vi "camera mjpeg.vi"(11 "CameraDevRef":T1) -> ()   [LabVIEW 2013]
uses:
  <vilib>/Rock Robotics/WPI/Camera/WPI_CameraDevRef.ctl
  <vilib>/Rock Robotics/WPI/Camera/WPI_CameraSettings Operations.ctl
  typedefs/fg_getset.ctl
  typedefs/vision/vision enable.ctl
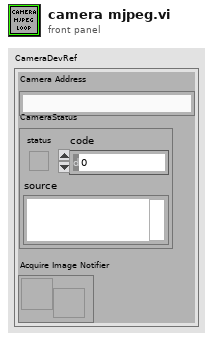
[diagram p1: front panel]
types:
  T1 = typedef "WPI_CameraDevRef.ctl" = cluster{"Camera Address":string, "CameraStatus":errorcluster, "Acquire Image Notifier":refnum<notifier>}
  T2 = typedef "WPI_CameraSettings Operations.ctl" = enum16{"Udate FPS", "Update Compression", "Update Size", "Update White Balance", "Update Brightness", "Update Sharpness", "Update Exposure", "Update Color Level", "Update Exp Priority", "Update Color Enable", "Update JPG", "Update MJPG", "Read and Clear", "Read", "Init"}
  T3 = typedef "vision enable.ctl" = enum16{"Enable", "Disable", "Stop"}
  T4 = typedef "fg_getset.ctl" = enum16{"Get", "Set"}
  T5 = typedef "WPI_CameraSettings Control.ctl" = cluster{"FPS":i32, "Compression":i32, "Size":i32, "White Balance":i32, "Brightness":i32, "Sharpness":i32, "Exposure":i32, "Color Level":i32, "Exposure Priority":i32, "Color Enable":i32, "JPG Loop":i32, "MJPG Loop":i32}
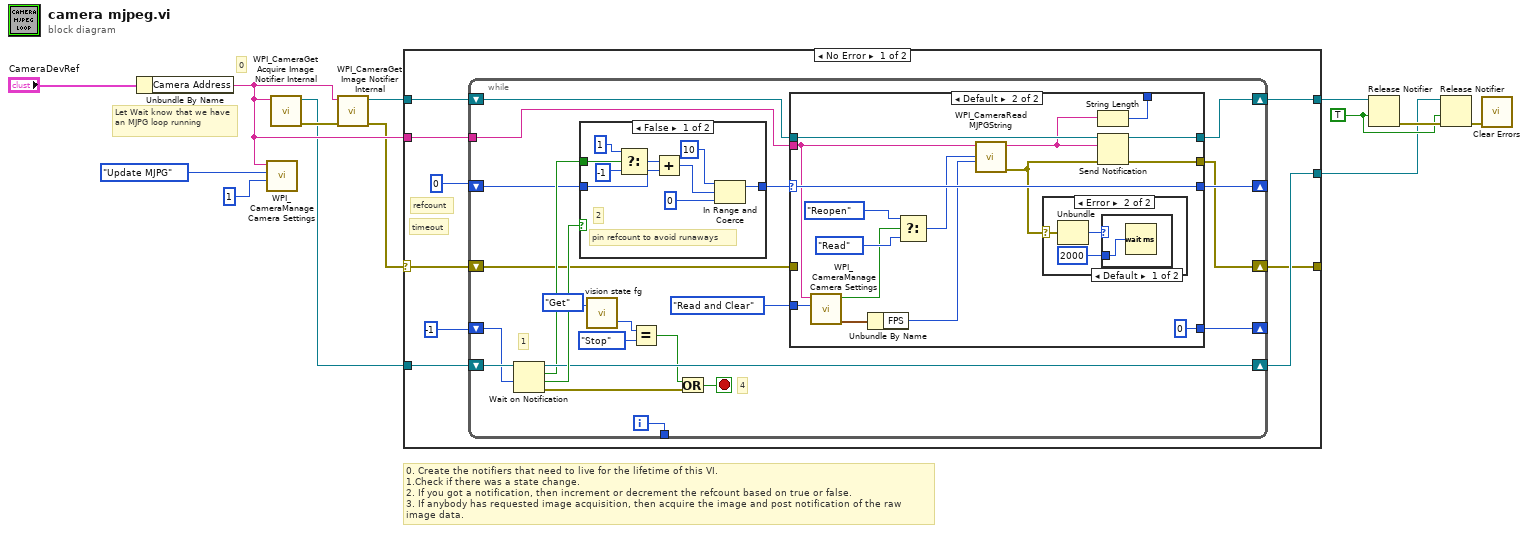
[diagram p0: block diagram]
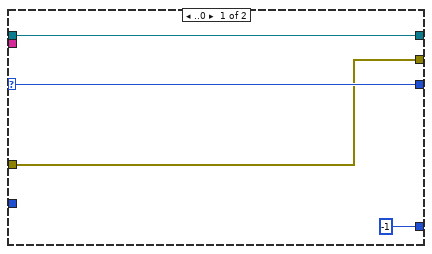
[diagram p2: hidden frame]
diagram:
  w4 = TRUE ("force destroy? (F)")
  # "Let Wait know that we have\nan MJPG loop running"
  # "0"
  # "0. Create the notifiers that need to live for the lifetime of this VI. \n1.Check if there was a state change.\n2. If you got a notification, then increment or decrement the refcount based on true or false.\n3. If anybody has requested image acquisition, then acquire the image and post notification of the raw image data."
  n1 = Unbundle By Name("CameraDevRef") -> ("Camera Address"=w12:string)
  n2 = call <vilib>:"WPI_CameraManage Camera Settings.vi"("Value"=1, "Operation"=WPI_CameraSettings_Operations."Update MJPG", "Camera IP"=w12) -> ()  [unwired: 7 in, 2 out]
  n3 = call <vilib>:"WPI_CameraGet Acquire Image Notifier Internal.vi"("Camera Address"=w12) -> ("error out"=w8:errorcluster, "Acquire Image Notifier"=w7:refnum<notifier>)  [unwired: 1 in, 8 out]
  n4 = call <vilib>:"WPI_CameraGet Image Notifier Internal.vi"("error in (no error)"=w8, "Camera Address"=w12) -> ("error out"=w5:errorcluster, "Image Notifier"=w3:refnum<notifier>)  [unwired: 8 out]
  n5 = case shown="No Error" w5 {
    selector: w5 -> [w15 w81]
    tunnel: w12 -> [w22 _]
    tunnel: w7 -> [w21 w79]
    tunnel: w3 -> [w19 w80]
    tunnel: [w17 w80] -> w1
    tunnel: [w16 w79] -> w2
    tunnel: [w14 w81] -> _
    frame No Error {
      # "timeout"
      # "refcount"
      n6 = while {
        shift-right: [w42] -> w16
        shift-left: w21 -> [w44]
        tunnel: w22 -> [w39]
        shift-right: [w31] -> _
        shift-left: 0 -> [w40]
        shift-right: [w37] -> w17
        shift-left: w19 -> [w38]
        shift-right: [w35] -> _
        shift-left: -1 -> [w36]
        shift-right: [w30] -> w14
        shift-left: w15 -> [w33]
        tunnel: [w28] -> _
        i -> [w28]
        stop <- w24 stop-if-true
        # "4"
        # "1"
        n7 = Wait on Notification(notifier=w44, timeout in ms (-1)=w36) -> (notifier out=w42:refnum<notifier>, notification=w41:bool, timed out?=w43:bool, error out=w34:errorcluster)  [unwired: 1 in, 1 out]
        n8 = case shown="False" w43 {
          tunnel: w41 -> [w77 _]
          tunnel: w40 -> [w73 w78]
          tunnel: [w69 w78] -> w32
          frame False {
            # "pin refcount to avoid runaways"
            # "2"
            n9 = Select(t=1, s=w77, f=-1) -> (s? t:f=w74:i32)
            n10 = Add(x=w74, y=w73) -> (x+y=w70:i32)
            n11 = In Range and Coerce(upper limit=10, x=w70, lower limit=0) -> (coerced(x)=w69:i32)  [unwired: 1 out]
          }
          frame True {
          }
        }
        n12 = call "vision state fg.vi"("Menu"=fg_getset."Get") -> ("State Out"=w26:T3)  [unwired: 1 in, 1 out]
        n13 = Equal?(x=w26, y=vision_enable."Stop") -> (x = y?=w23:bool)
        n14 = Or(x=w23, y=w34) -> (x .or. y?=w24:bool)
        n15 = case shown="Default" w32 {
          selector: w32 -> [w47 w61]
          tunnel: w39 -> [_ w49]
          tunnel: w38 -> [w48 w64]
          tunnel: [w48 w63] -> w37
          tunnel: [-1 0] -> w35
          tunnel: w33 -> [w45 _]
          tunnel: [w47 w61] -> w31
          tunnel: [w45 w60] -> w30
          tunnel: [_ w54] -> _
          tunnel: WPI_CameraSettings_Operations."Read and Clear" ("Operation") -> [_ w50]
          frame ..0 {
          }
          frame Default {
            n16 = call <vilib>:"WPI_CameraManage Camera Settings.vi"("Operation"=w50, "Camera IP"=w49) -> ("Values"=w52:T5, "Changed"=w53:bool)  [unwired: 8 in]
            n17 = Unbundle By Name(w52) -> ("FPS"=w51:i32)
            n18 = Select(t=enum16{"Read", "Reopen", "Close"}."Reopen" ("Operation"), s=w53, f=enum16{"Read", "Reopen", "Close"}."Read" ("Operation")) -> (s? t:f=w56:enum16{"Read", "Reopen", "Close"})
            n19 = call <vilib>:"WPI_CameraRead MJPGString.vi"("fps"=w51, "Operation"=w56, "address"=w49) -> ("error out"=w59:errorcluster, "Raw Image Data"=w55:string)  [unwired: 7 in]
            n20 = case shown="Error" w59 {
              selector: w59 -> [_ w67]
              frame No Error {
              }
              frame Error {
                n21 = Unbundle(w67) -> ("code"=w66:i32)  [unwired: 2 out]
                n22 = case shown="Default" w66 {
                  tunnel: u32 2000 ("milliseconds to wait") -> [w68 _]
                  frame Default {
                    n23 = Wait (ms)(milliseconds to wait=w68) -> ()  [unwired: 1 out]
                  }
                  frame 56 {
                  }
                }
              }
            }
            n24 = String Length(string=w55) -> (length=w54:i32)
            n25 = Send Notification(notification=w55, notifier=w64, error in (no error)=w59) -> (notifier out=w63:refnum<notifier>, error out=w60:errorcluster)
          }
        }
      }
    }
    frame Error {
    }
  }
  n26 = Release Notifier(notifier=w1, force destroy? (F)=w4) -> (error out=w9:errorcluster)  [unwired: 1 in, 2 out]
  n27 = Release Notifier(notifier=w2, force destroy? (F)=w4, error in (no error)=w9) -> (error out=w6:errorcluster)  [unwired: 2 out]
  n28 = call <vilib>:"Clear Errors.vi"("error in (no error)"=w6) -> ()  [unwired: 7 out]
